vi "Listbox_allTimesweeps.vi"(2 "new array":dbl[][](array[numeric])) -> (0 "New listbox":string[](array[string]), 1 "output array":string[](array[string]))   [LabVIEW 2018]
panel:
  out "concatenated string":string
  out "Numeric":i32
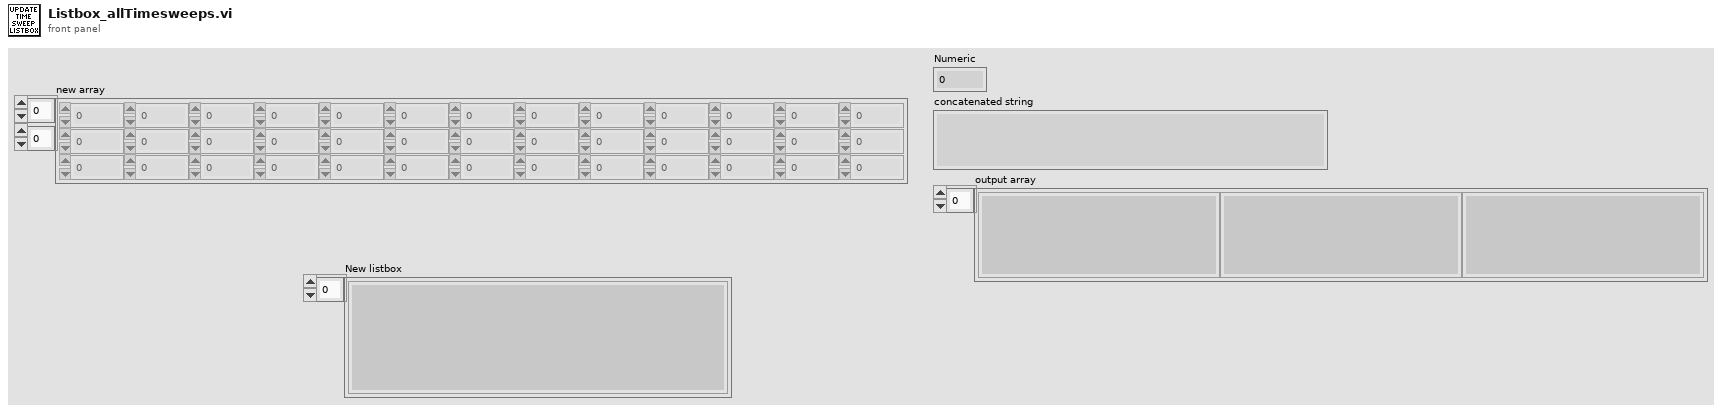
[diagram p1: front panel]
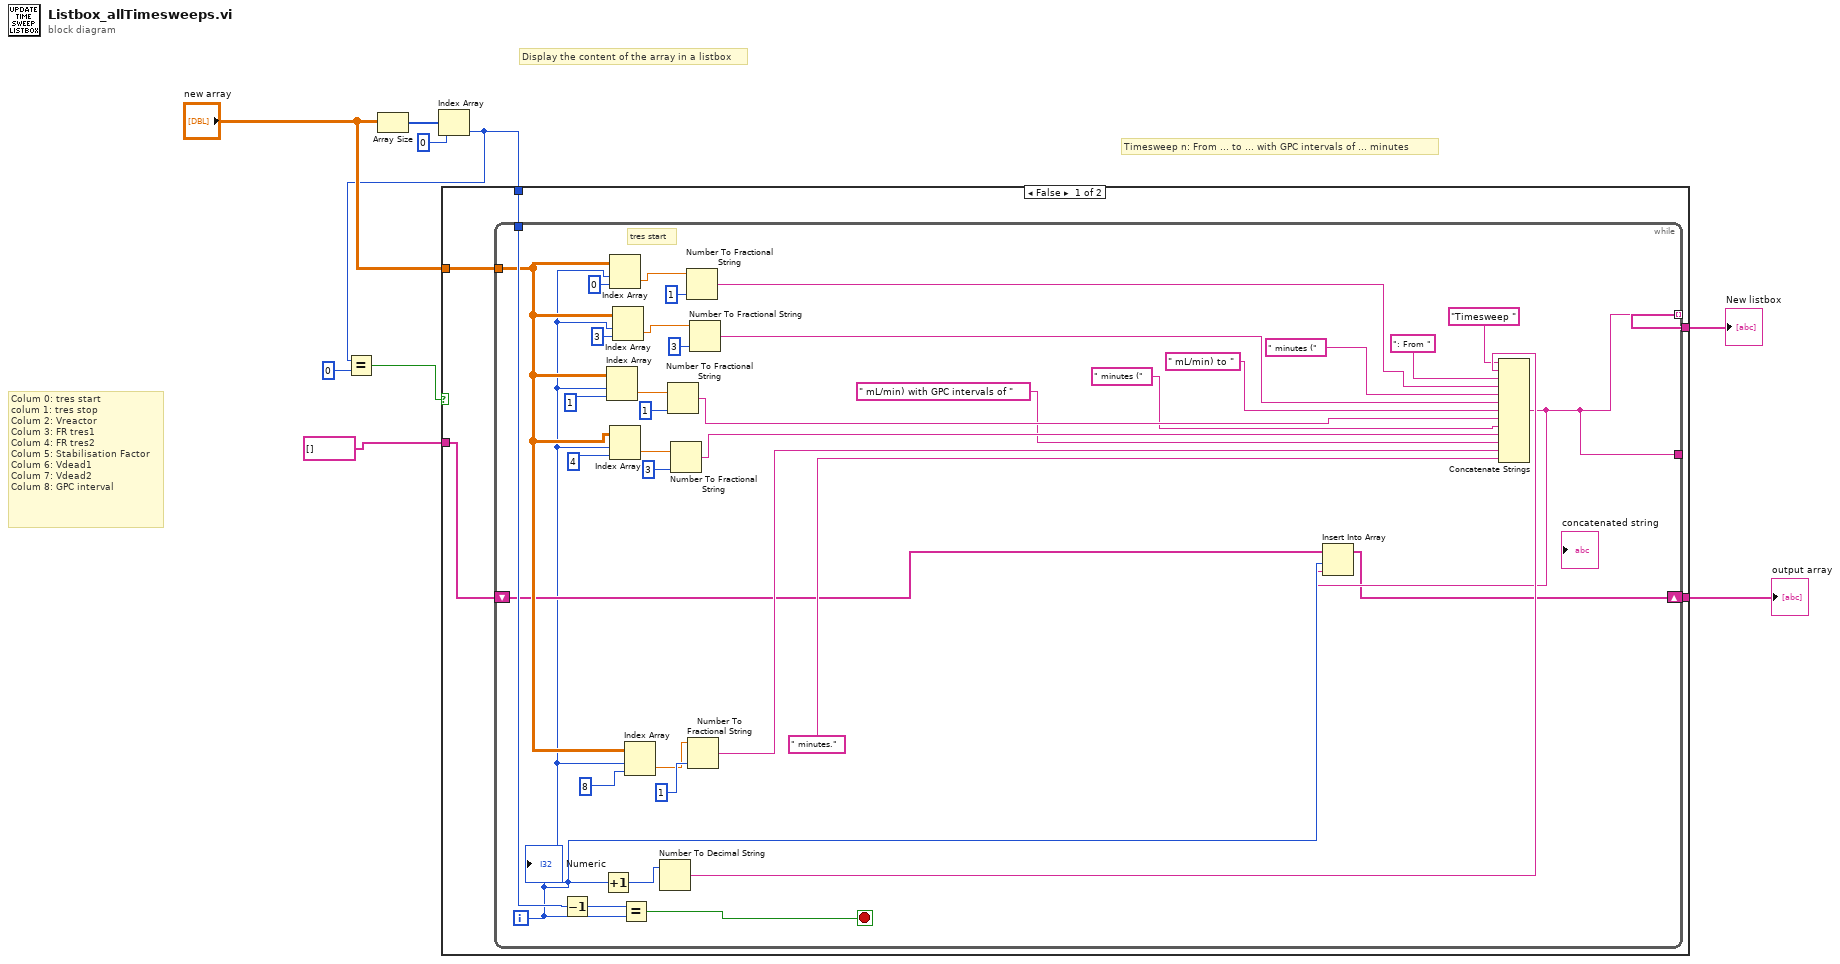
[diagram p0: block diagram]
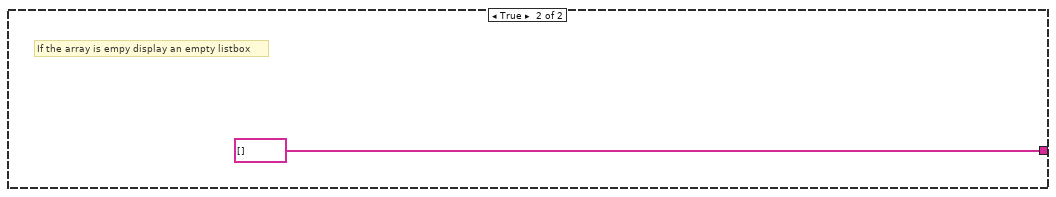
[diagram p2: hidden frame]
diagram:
  # "Timesweep n: From ... to ... with GPC intervals of ... minutes"
  # "Colum 0: tres start\ncolum 1: tres stop\nColum 2: Vreactor\nColum 3: FR tres1\nColum 4: FR tres2\nColum 5: Stabilisation Factor\nColum 6: Vdead1\nColum 7: Vdead2\nColum 8: GPC interval"
  # "Display the content of the array in a listbox"
  n1 = Array Size(array="new array") -> (size(s)=w9:i32[])
  n2 = Index Array(array=w9, index=0) -> (element=w5:i32)
  n3 = Equal?(x=w5, y=0) -> (x = y?=w3:bool)
  n4 = case shown="False" w3 {
    tunnel: "new array" -> [w14 _]
    tunnel: w5 -> [w13 _]
    tunnel: [w12 string[] []] -> w6
    tunnel: string[] [] -> [w11 _]
    tunnel: [w10 _] -> w1
    frame False {
      n5 = while {
        tunnel: w14 -> [w23]
        tunnel: w13 -> [w45]
        tunnel: [w16] -> w12 mode=indexing
        tunnel: [w16] -> _
        shift-right: [w15] -> w10
        shift-left: w11 -> [w18]
        i -> [w17]
        stop <- w51 stop-if-true
        # "tres start"
        n6 = Decrement(x=w45) -> (x-1=w46:i32)
        n7 = Increment(x=w17) -> (x+1=w50:i32)
        n8 = Index Array(array=w23, index (row)=w17, index (col)=1 ("disabled index (col)")) -> (element=w43:dbl)
        n9 = Index Array(array=w23, index (row)=w17, index (col)=0 ("disabled index (col)")) -> (element=w48:dbl)
        n10 = Index Array(array=w23, index (row)=w17, index (col)=4 ("disabled index (col)")) -> (element=w25:dbl)
        n11 = Index Array(array=w23, index (row)=w17, index (col)=3 ("disabled index (col)")) -> (element=w31:dbl)
        n12 = Equal?(x=w46, y=w17) -> (x = y?=w51:bool)
        n13 = Index Array(array=w23, index (row)=w17, index (col)=8 ("disabled index (col)")) -> (element=w40:dbl)
        n14 = Number To Decimal String(number=w50) -> (decimal integer string=w38:string)  [unwired: 1 in]
        n15 = Number To Fractional String(number=w43, precision (6)=i16 1) -> (F-format string=w22:string)  [unwired: 2 in]
        n16 = Number To Fractional String(number=w25, precision (6)=i16 3) -> (F-format string=w20:string)  [unwired: 2 in]
        n17 = Number To Fractional String(number=w48, precision (6)=i16 1) -> (F-format string=w34:string)  [unwired: 2 in]
        n18 = Number To Fractional String(number=w40, precision (6)=i16 1) -> (F-format string=w27:string)  [unwired: 2 in]
        n19 = Number To Fractional String(number=w31, precision (6)=i16 3) -> (F-format string=w29:string)  [unwired: 2 in]
        n20 = Concatenate Strings("Timesweep " ("string"), w38, ": From " ("string"), w34, " minutes (" ("string"), w29, " mL/min) to " ("string"), w22, " minutes (" ("string"), w20, " mL/min) with GPC intervals of " ("string"), w27, " minutes." ("string")) -> (w16:string)
        n21 = Insert Into Array(array=w18, index=w17, new element=w16) -> (w15:string[])
        "Numeric" <- w17
      }
    }
    frame True {
      # "If the array is empy display an empty listbox"
    }
  }
  "New listbox" <- w6
  "output array" <- w1
